vi "CAN 6 TalonSRX Motor Set Value.vi"(6 "Control Mode":T1 items=["PercentOutput"=0, "Position"=1, "Velocity"=2, "Current"=3, "Follower"=5, "MotionProfile"=6, "MotionMagic"=7, "MotionMagicArc"=8, "MotionProfileArc"=10, "Disabled"=15], 7 "Velocity Offset":dbl, 9 "Right Power":dbl, 10 "Left Power":dbl, 11 "Drivetrain":T2) -> ()   [LabVIEW 2017]
uses:
  TalonSRX6Motor.ctl
  <vilib>/Rock Robotics/WPI/MotorControl/WPI_MotorControlDeviceRef.ctl
  <vilib>/Rock Robotics/WPI/MotorControl/WPI_MotorControlType.ctl
  <vilib>/Rock Robotics/SystemInterfaces/DIO/FPGA_DIOPWMChannel.ctl
  <vilib>/Rock Robotics/WPI/PWM/WPI_PWMDeadband.ctl
  <vilib>/Rock Robotics/SystemInterfaces/DIO/FPGA_DIOChannel.ctl
  <vilib>/Rock Robotics/WPI/ThirdParty/Phoenix-LabVIEW/Motor Controller/Controls/CTRE_Phoenix_MotorControl_ControlMode.ctl
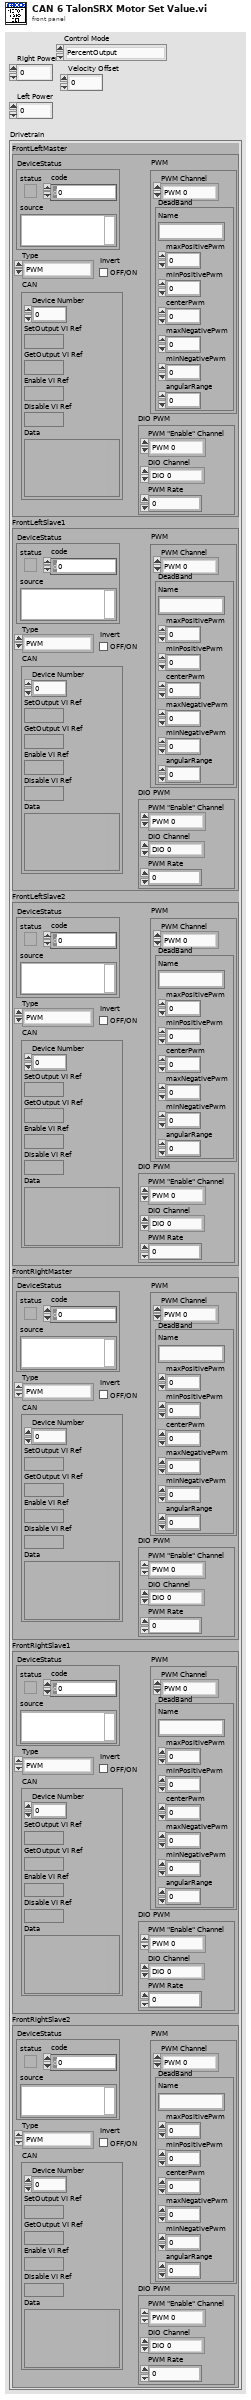
[diagram p1: front panel]
types:
  T1 = typedef "CTRE_Phoenix_MotorControl_ControlMode.ctl" = u16
  T2 = typedef "TalonSRX6Motor.ctl" = cluster{"FrontLeftMaster":T3, "FrontLeftSlave1":T3, "FrontLeftSlave2":T3, "FrontRightMaster":T3, "FrontRightSlave1":T3, "FrontRightSlave2":T3}
  T3 = typedef "WPI_MotorControlDeviceRef.ctl" = cluster{"DeviceStatus":errorcluster, "Type":T4, "PWM":cluster{"PWM Channel":T5, "DeadBand":T6}, "CAN":cluster{"Device Number":u8, "SetOutput VI Ref":variant, "GetOutput VI Ref":variant, "Enable VI Ref":variant, "Disable VI Ref":variant, "Data":variant}, "Invert":bool, "DIO PWM":cluster{"PWM \"Enable\" Channel":T5, "DIOChannel":T7, "PWM Rate":dbl}}
  T4 = typedef "WPI_MotorControlType.ctl" = enum16{"PWM", "CAN", "DIO PWM"}
  T5 = typedef "FPGA_DIOPWMChannel.ctl" = enum8{"PWM 0", "PWM 1", "PWM 2", "PWM 3", "PWM 4", "PWM 5", "PWM 6", "PWM 7", "PWM 8", "PWM 9", "PWM MXP 0", "PWM MXP 1", "PWM MXP 2", "PWM MXP 3", "PWM MXP 4", "PWM MXP 5", "PWM MXP 6", "PWM MXP 7", "PWM MXP 8", "PWM MXP 9", "Invalid"}
  T6 = typedef "WPI_PWMDeadband.ctl" = cluster{"Name":string, "maxPositivePwm":i32, "minPositivePwm":i32, "centerPwm":i32, "maxNegativePwm":i32, "minNegativePwm":i32, "angularRange":u16}
  T7 = typedef "FPGA_DIOChannel.ctl" = enum8{"DIO 0", "DIO 1", "DIO 2", "DIO 3", "DIO 4", "DIO 5", "DIO 6", "DIO 7", "DIO 8", "DIO 9", "DIO MXP 0", "DIO MXP 1", "DIO MXP 2", "DIO MXP 3", "DIO MXP 4", "DIO MXP 5", "DIO MXP 6", "DIO MXP 7", "DIO MXP 8", "DIO MXP 9", "DIO MXP 10", "DIO MXP 11", "DIO MXP 12", "DIO MXP 13", "DIO MXP 14", "DIO MXP 15", "SPI Port CS1", "SPI Port CS2", "SPI Port CS3", "SPI Port MISO", "SPI Port MOSI", "Invalid"}
  T8 = enum16{"DemandType_Neutral", "DemandType_AuxPID", "DemandType_ArbitraryFeedForward"}
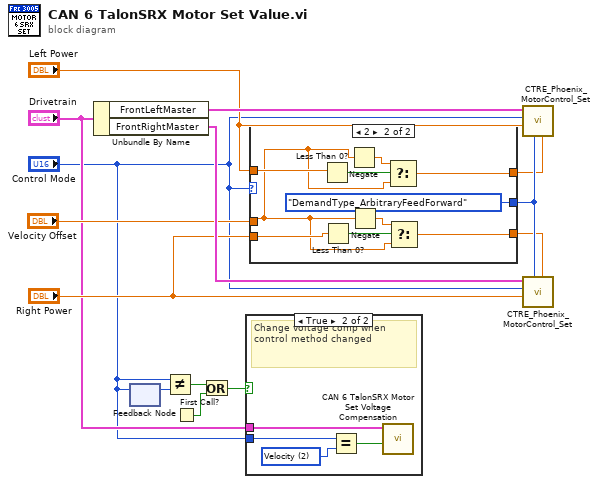
[diagram p0: block diagram]
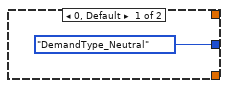
[diagram p3: hidden frame]
diagram:
  n1 = Unbundle By Name("Drivetrain") -> ("FrontLeftMaster"=w13:T3, "FrontRightMaster"=w14:T3)
  n2 = feedback-in #1("Control Mode") -> ()
  n3 = feedback #1() -> (w2:T1)  [unwired: 1 in]
  n4 = Not Equal?(x="Control Mode", y=w2) -> (x != y?=w5:bool)
  n5 = First Call?() -> (First Call?: T/F=w3:bool)
  n6 = Or(x=w5, y=w3) -> (x .or. y?=w4:bool)
  n7 = case shown="True" w4 {
    tunnel: "Drivetrain" -> [_ w18]
    tunnel: "Control Mode" -> [_ w17]
    frame False {
    }
    frame True {
      w16 = T1 2 items=["PercentOutput"=0, "Position"=1, "Velocity"=2, "Current"=3, "Follower"=5, "MotionProfile"=6, "MotionMagic"=7, "MotionMagicArc"=8, "MotionProfileArc"=10, "Disabled"=15] ("y")
      # "Change voltage comp when control method changed"
      n8 = Equal?(x=w17, y=w16) -> (x = y?=w15:bool)
      n9 = call "CAN 6 TalonSRX Motor Set Voltage Compensation.vi"("Enable Voltage Compensation? (F)"=w15, "TalonSRX6MotorRef"=w18) -> ()  [unwired: 9 in, 1 out]
    }
  }
  n10 = case shown="2" "Control Mode" {
    tunnel: [T8."DemandType_Neutral" ("DemandType") T8."DemandType_ArbitraryFeedForward" ("DemandType")] -> w10
    tunnel: "Right Power" -> [_ w22]
    tunnel: "Left Power" -> [_ w26]
    tunnel: "Velocity Offset" -> [_ w21]
    tunnel: [_ w25] -> w8
    tunnel: [_ w20] -> w7
    frame 0, Default {
    }
    frame 2 {
      n11 = Less Than 0?(x=w26) -> (x < 0?=w28:bool)
      n12 = Less Than 0?(x=w22) -> (x < 0?=w23:bool)
      n13 = Negate(x=w21) -> (-x=w27:dbl)
      n14 = Negate(x=w21) -> (-x=w24:dbl)
      n15 = Select(t=w27, s=w28, f=w21) -> (s? t:f=w25:dbl)
      n16 = Select(t=w24, s=w23, f=w21) -> (s? t:f=w20:dbl)
    }
  }
  n17 = call <vilib>:"CTRE_Phoenix_MotorControl_Set.vi"("Demand1"=w8, "DemandType"=w10, "Output"="Left Power", "Control Mode"="Control Mode", "PhoenixMotorControlDevRef"=w13) -> ()  [unwired: 5 in, 2 out]
  n18 = call <vilib>:"CTRE_Phoenix_MotorControl_Set.vi"("Demand1"=w7, "DemandType"=w10, "Output"="Right Power", "Control Mode"="Control Mode", "PhoenixMotorControlDevRef"=w14) -> ()  [unwired: 5 in, 2 out]
